vi "ManualWriteFile.vi"(8 "ErrorIn":errorcluster caption="Error In", 10 "DataToWrite":T1[](array[typedef])=[{"ThisNavigationName"="root", "ButtonLabel"="btn 1", "Caption"="Doe iets", "Tooltip"="iets", "EnabledExpression"="Enable", "Actions"=[{"ActionType"="Call", "TargetObject"="TestUI", "Parameter"="doe", "WaitUntilDone"=TRUE}], "NextNavigationName"="Level 1"}, {"ThisNavigationName"="root", "ButtonLabel"="btn 12", "Caption"="Exit", "Tooltip"="Stop the app", "EnabledExpression"="Enable", "Actions"=[{"ActionType"="Call", "TargetObject"="ButtonBar", "Parameter"="Exit", "WaitUntilDone"=FALSE}], "NextNavigationName"="root"}, {"ThisNavigationName"="Level 1", "ButtonLabel"="btn 2", "Caption"="tweede", "Tooltip"="", "EnabledExpression"="Enable", "Actions"=[], "NextNavigationName"="Level 2"}, {"ThisNavigationName"="Level 1", "ButtonLabel"="btn 12", "Caption"="Back", "Tooltip"="", "EnabledExpression"="Enable", "Actions"=[], "NextNavigationName"="root"}, {"ThisNavigationName"="Level 2", "ButtonLabel"="btn 3", "Caption"="derde", "Tooltip"="", "EnabledExpression"="Enable", "Actions"=[], "NextNavigationName"="Level 1"}], 11 "FilePath":path=path "C:/Users/fambr/OneDrive/Documenten/LabVIEW Projecten/InterfaceApplicationDesign/ApplicationConfiguration/Default/ButtonBarDefinition.json") -> (0 "ErrorOut":errorcluster caption="Error Out")   [LabVIEW 2021, in "ButtonCollection.lvclass"]
uses:
  ButtonCollection.lvclass
  ButtonDefinition.ctl
  ButtonCollection.lvclass/ButtonCollection.ctl
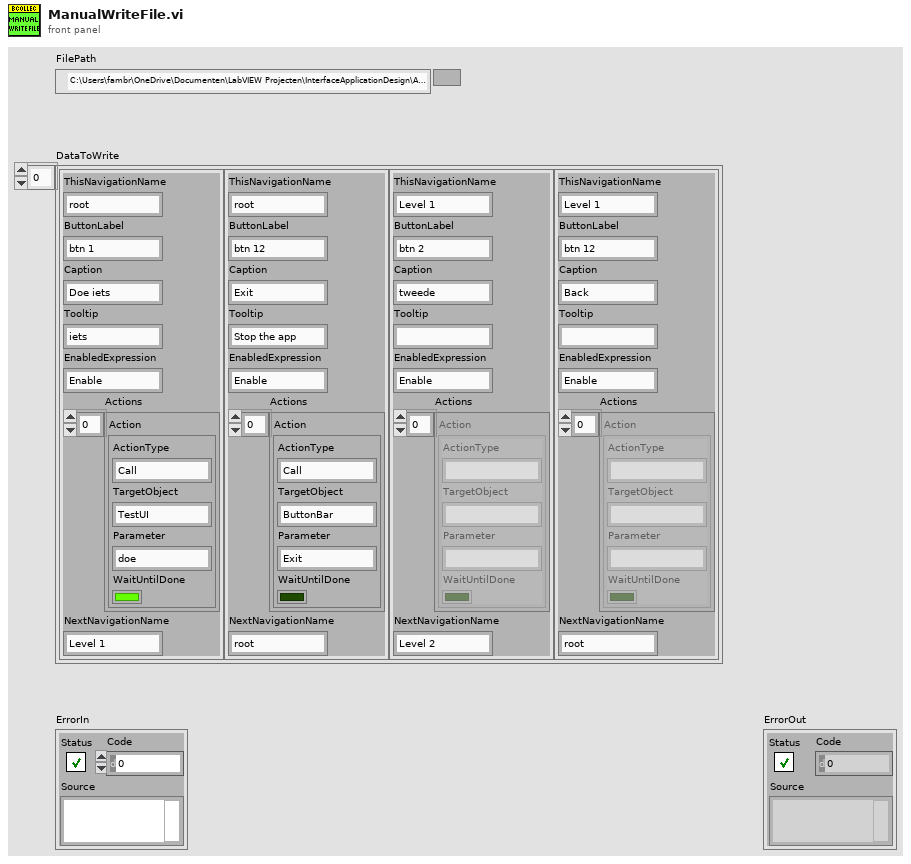
[diagram p1: front panel]
types:
  T1 = typedef "ButtonCollection.lvclass/ButtonDefinition.ctl" = cluster{"ThisNavigationName":string, "ButtonLabel":string, "Caption":string, "Tooltip":string, "EnabledExpression":string, "Actions":cluster{"ActionType":string, "TargetObject":string, "Parameter":string, "WaitUntilDone":bool}[], "NextNavigationName":string}
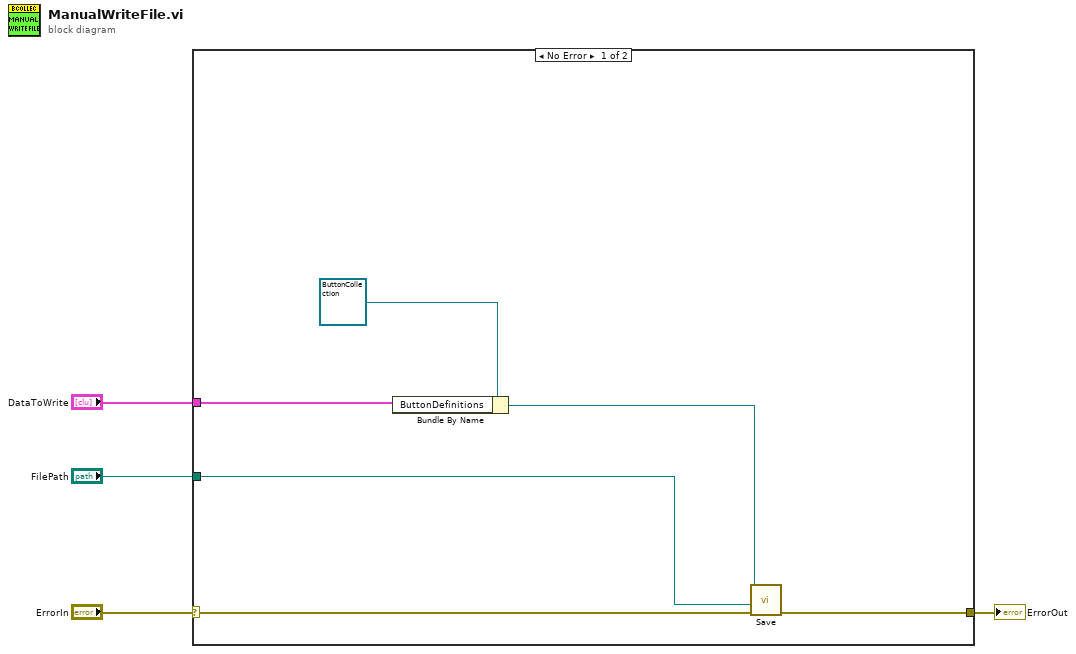
[diagram p0: block diagram]
diagram:
  n1 = case shown="No Error" "ErrorIn" {
    selector: "ErrorIn" -> [w10 w11]
    tunnel: [w9 w11] -> w3
    tunnel: "DataToWrite" -> [w7 _]
    tunnel: "FilePath" -> [w5 _]
    frame No Error {
      n2 = Bundle By Name(cluster=refnum<class "ButtonCollection.lvclass"> refnum ("TryButton.lvlib:ButtonCollection"), "ButtonDefinitions"=w7) -> (w6:refnum<class "ButtonCollection.lvclass">)
      n3 = call "Save.vi"("ErrorIn"=w10, "Path"=w5, "ObjectIn"=w6) -> ("ErrorOut"=w9:errorcluster)  [unwired: 7 in, 1 out]
    }
    frame Error {
    }
  }
  "ErrorOut" <- w3
